vi "Camera.Simulated.GetDependencies.vi"(8 "error in (no error)":errorcluster, 11 "Camera.Simulated":refnum<class "Camera.Simulated.lvclass">) -> (0 "error out":errorcluster, 2 "Dependencies":T1, 3 "Camera.Simulated":refnum<class "Camera.Simulated.lvclass">)   [LabVIEW 2013, in "Camera.Simulated.lvclass"]
doc: "---------------------------------------------------------------\nJKI State Machine Objects™\nhttp://jki.net/state-machine-objects/\nCopyright (C) 2005-2015, JKI <info@jki.net>\nALL RIGHTS RESERVEDJKI State Machine Objects (SMO) 1.0.0.5\nJKI - JKI\nCopyright (c) 2016, JKI"
uses:
  Camera.Simulated.lvclass
  Dependencies--Cluster.ctl
  CircularBuffer.ImageData/CircularBuffer.ImageData.lvclass
panel:
  # "For instructions on how to use the JKI State Machine Objects, examples and video tutorials, visit:\nhttp://jki.net/state-machine-objects/\n\nJKI State Machine Objects™\nhttp://jki.net/state-machine-objects/\nCopyright (C) 2005-2015, JKI <info@jki.net>\nALL RIGHTS RESERVED"
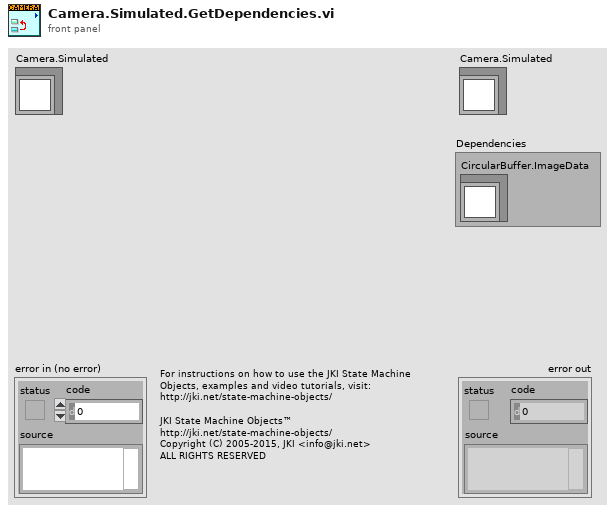
[diagram p1: front panel]
types:
  T1 = typedef "Camera.Simulated.lvclass/Dependencies--Cluster.ctl" = cluster{"CircularBuffer.ImageData":refnum<class "CircularBuffer.ImageData.lvclass">}
  T2 = typedef "Camera.Simulated.lvclass/PrivateData--Ref.ctl" = refnum<data-value>
  T3 = typedef "Camera.Simulated.lvclass/PrivateData--Cluster.ctl" = cluster{"Dependencies":T1, "Configuration":T4}
  T4 = typedef "Camera.Simulated.lvclass/Configuration--CLuster.ctl" = cluster{"Simulated Images Folder":path, "filetype":string}
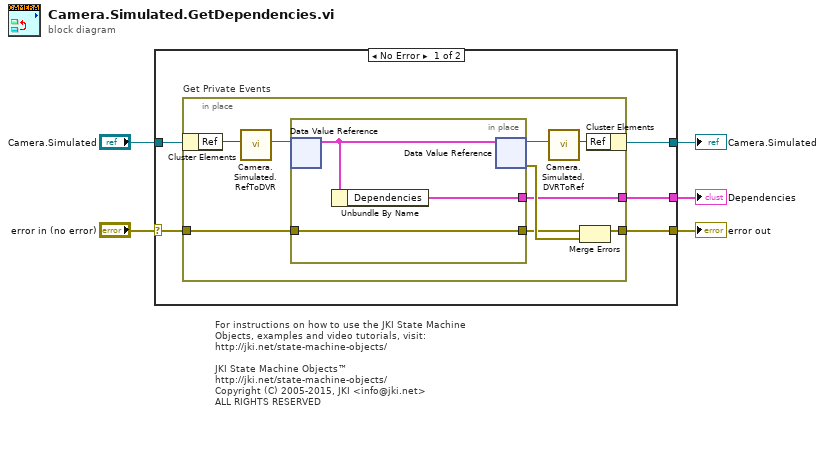
[diagram p0: block diagram]
diagram:
  # "For instructions on how to use the JKI State Machine Objects, examples and video tutorials, visit:\nhttp://jki.net/state-machine-objects/\n\nJKI State Machine Objects™\nhttp://jki.net/state-machine-objects/\nCopyright (C) 2005-2015, JKI <info@jki.net>\nALL RIGHTS RESERVED"
  n1 = case shown="No Error" "error in (no error)" {
    selector: "error in (no error)" -> [w9 w23]
    tunnel: "Camera.Simulated" -> [w10 w24]
    tunnel: [w8 w23] -> w4
    tunnel: [w7 w24] -> w3
    tunnel: [w6 _] -> w1
    frame No Error {
      n2 = in-place "Get Private Events" {
        in-place-border: w9 -> [w19]
        in-place-border: [w16] -> w8
        in-place-border: [w15] -> w6
        n3 = in-place-cluster #1(w10) -> ("Ref"=w14:u32)
        n4 = call "Camera.Simulated.RefToDVR.vi"("Ref"=w14) -> ("Ref"=w13:T2)  [unwired: 10 in]
        n5 = in-place {
          in-place-border: w19 -> [w21]
          in-place-border: [w21] -> w17
          in-place-border: [w20] -> w15
          n6 = in-place-dvr #2(w13) -> (w22:T3)  [unwired: 1 out]
          n7 = Unbundle By Name(w22) -> ("Dependencies"=w20:T1)
          n8 = in-place-dvr #2(w22) -> (w12:T2, w18:errorcluster)
        }
        n9 = call "Camera.Simulated.DVRToRef.vi"("Ref"=w12) -> ("Ref"=w11:u32)  [unwired: 10 in]
        n10 = Merge Errors(w17, w18) -> (w16:errorcluster)
        n11 = in-place-cluster #1("Ref"=w11) -> (w7:refnum<class "Camera.Simulated.lvclass">)
      }
    }
    frame Error {
    }
  }
  "error out" <- w4
  "Camera.Simulated" <- w3
  "Dependencies" <- w1
